vi "Write Control.vi"(5 "High Address":u32 format="%08x", 7 "Base Address":u32 format="%08x", 9 "Data":u32 format="%08x", 11 "Address":u32 format="%08x") -> (0 "Error":bool)   [LabVIEW 2011]
uses:
  Globals.vi
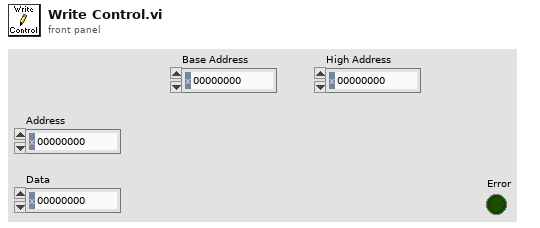
[diagram p1: front panel]
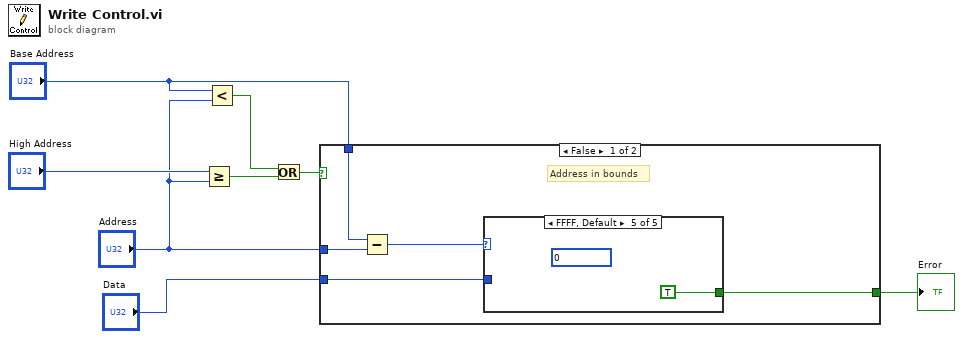
[diagram p0: block diagram]
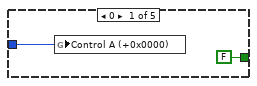
[diagram p2: hidden frame]
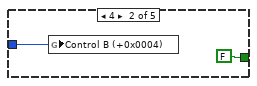
[diagram p3: hidden frame]
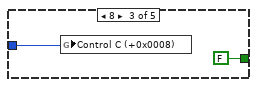
[diagram p4: hidden frame]
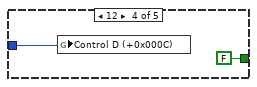
[diagram p5: hidden frame]
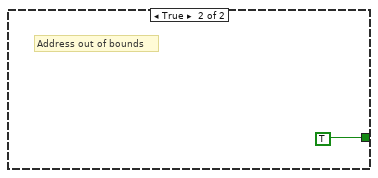
[diagram p6: hidden frame]
diagram:
  n1 = Greater Or Equal?(x="High Address", y="Address") -> (x >= y?=w7:bool)
  n2 = Less?(x="Base Address", y="Address") -> (x < y?=w6:bool)
  n3 = Or(x=w6, y=w7) -> (x .or. y?=w8:bool)
  n4 = case shown="False" w8 {
    tunnel: [w12 TRUE ("Error")] -> w4
    tunnel: "Address" -> [w11 _]
    tunnel: "Base Address" -> [w10 _]
    tunnel: "Data" -> [w9 _]
    frame False {
      # "Address in bounds"
      n5 = Subtract(x=w10, y=w11) -> (x-y=w13:u32)
      n6 = case shown="FFFF, Default" w13 {
        tunnel: [FALSE ("Error") FALSE ("Error") FALSE ("Error") FALSE ("Error") TRUE ("Error")] -> w12
        tunnel: w9 -> [w14 w16 w18 w20 _]
        frame 0 {
          n7 = global write "Globals.vi" "Control A (+0x0000)"(w14) -> ()
        }
        frame 4 {
          n8 = global write "Globals.vi" "Control B (+0x0004)"(w16) -> ()
        }
        frame 8 {
          n9 = global write "Globals.vi" "Control C (+0x0008)"(w18) -> ()
        }
        frame 12 {
          n10 = global write "Globals.vi" "Control D (+0x000C)"(w20) -> ()
        }
        frame 65535, Default {
          (unwired) 0 ("Data")
        }
      }
    }
    frame True {
      # "Address out of bounds"
    }
  }
  "Error" <- w4
